vi "WriteRngSeed.vi"(8 "error in":errorcluster, 11 "seed":i32) -> (0 "error out":errorcluster)   [LabVIEW 2020, in "OpenLvVision_OpenCv.lvlib"]
doc: "Sets state of default random number generator."
uses:
  OpenLvVision_OpenCv.lvlib
  Dlls/OlvOpenCvWrapper.dll
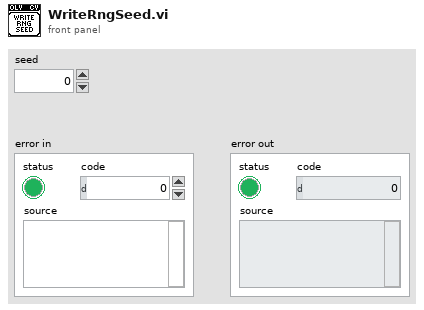
[diagram p1: front panel]
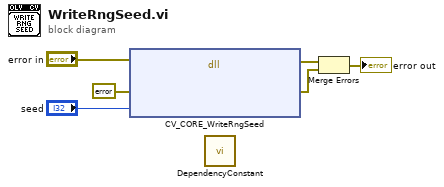
[diagram p0: block diagram]
diagram:
  n1 = dll-call lib="C:/Users/lukas/Downloads/OpenLvVision_OpenCv/SourceCode/LabView/OpenLvVision_OpenCv/Dlls/OlvOpenCvWrapper.dll" fn="CV_CORE_WriteRngSeed"(error in="error in", "Error"=errorcluster {"status"=FALSE, "code"=0, "source"=""} ("error constant"), "seed"="seed") -> (error out=w5:errorcluster, "Error"=w1:errorcluster)  [unwired: 4 in, 1 out]
  n2 = call "DependencyConstant.vi"() -> ()  [unwired: 12 in]
  n3 = Merge Errors(w5, w1) -> (→"error out":errorcluster)
